vi "svx_Orbit SC Menu.vi"(6 "Run Mode?":bool, 7 "State":T2={"X Scale"={"Name"="Horizontal", "FString"="%#.2g", "Major Color"=16777238, "Minor Color"=16777216, "Scale Visible"=TRUE, " Label Visible"=TRUE, "Grid Style"=1}, "Y Scale"={"Name"="Vertical", "FString"="%#.2g", "Major Color"=16777238, "Minor Color"=16777216, "Scale Visible"=TRUE, " Label Visible"=TRUE, "Grid Style"=1}, "Plot"={"Point Style"=0, "Line Width"=0, "Line Style"=0, "Plot Color"=9727, "Point/fill"=0}, "Arrow/Crosshair Color"=9727, "Tacho Point Color"=16711680, "Container Bounds"={"Width"=563, "Height"=294}, "Axis Maximum"=10.0, "Probe Angles"={"Angle X"=0.0, "Angle Y"=1.5707963267948966}, "Background Color"=16777226, "Cursor"={"Cursor Point Style"=13, "Cursor Style"=4, "Cursor Line Width"=1, "Cursor Line Style"=0, "Cursor Color"=9727, "Cursor Name Visible"=TRUE, "Cursor Visible"=TRUE, "Cursor Position"={"X"=0.0, "Y"=0.0}, "Cursor Index"=0, "Cursor Lock"=FALSE}, "Elliptical Info"=[], "Legend Visible"=TRUE, "Scale Range Change"=refnum, "Strings[]"={"Custom pair name"=FALSE, "Row Strings []"=[], "Column Strings []"=[]}, "Index"=[{"pair index"=0, "order index"=0}], " Parents Tags"=[], "Children Tags"=[], "Open?"=[], "Label"="", "Legend Width"=120, "Pair Strings Changed?"=FALSE, "Size"=[], "Legend Background"=16777226, "Legend Font"=16777222, "Cursor Release"=refnum, "Autoscale"=TRUE, "Precession Direction"=[], "Item Width"=0, "User Pair Strings []"=[], "Users Order Strings []"=[], "Autoscale Once"=TRUE, "Property Write"=refnum} {"Index"."order index" min=0; "Index"."pair index" min=0; "Axis Maximum" min=0.0}, 10 "Refnum":refnum<vi>, 11 "MenuRef":refnum<k9>) -> ()   [LabVIEW 2017, in "SVX Orbit.xctl"]
uses:
  <vilib>/addons/_XControls/Orbit Plot/SVX Orbit.xctl
  <vilib>/addons/_XControls/Orbit Plot/subVIs/svx_Orbit Internal State.ctl
  <vilib>/addons/_XControls/Orbit Plot/subVIs/svx_Orbit Bounds.ctl
panel:
  in  "Run-time\nnew menu":T1(array[cluster])=[{"menu tag"="APP_SC_VISIBLE_ITEMS", "item names"="Plot Legend", "item tags"="USER_SC_SELECTOR", ""}, {"menu tag"="APP_SC_VISIBLE_ITEMS", "item names"="-", "item tags"="APP_SC_SEPERATOR_3", "USER_SC_SELECTOR"}, {"menu tag"="APP_SC_VISIBLE_ITEMS", "item names"="X Scale", "item tags"="USER_SC_X_SCALE", "APP_SC_SEPERATOR_3"}, {"menu tag"="APP_SC_VISIBLE_ITEMS", "item names"="Y Scale", "item tags"="USER_SC_Y_SCALE", "USER_SC_X_SCALE"}, {"menu tag"="APP_SC_VISIBLE_ITEMS", "item names"="-", "item tags"="APP_SC_SEPERATOR", "USER_SC_Y_SCALE"}, {"menu tag"="APP_SC_VISIBLE_ITEMS", "item names"="Cursor", "item tags"="USER_SC_CURSOR", "APP_SC_SEPERATOR"}, {"menu tag"="APP_SC_VISIBLE_ITEMS", "item names"="Cursor Info", "item tags"="USER_SC_CURSORINFO", "USER_SC_CURSOR"}, {"menu tag"="APP_SC_VISIBLE_ITEMS", "item names"="Lock Cursor Info Position", "item tags"="USER_SC_LOCK", "USER_SC_CURSORINFO"}, {"menu tag"="", "item names"="Autoscale", "item tags"="USER_SC_AUTOSCALE", ""}]
  in  "Edit-time\nnew menu":T1(array[cluster])=[{"menu tag"="USER_SC_VISIBLE_ITEMS", "item names"="Label", "item tags"="USER_SC_LABEL", ""}, {"menu tag"="USER_SC_VISIBLE_ITEMS", "item names"="Caption", "item tags"="USER_SC_CAPTION", "USER_SC_LABEL"}, {"menu tag"="USER_SC_VISIBLE_ITEMS", "item names"="-", "item tags"="APP_SC_SEPERATOR", "USER_SC_CAPTION"}, {"menu tag"="USER_SC_VISIBLE_ITEMS", "item names"="Plot Legend", "item tags"="USER_SC_SELECTOR", "APP_SC_SEPERATOR"}, {"menu tag"="USER_SC_VISIBLE_ITEMS", "item names"="-", "item tags"="APP_SC_SEPERATOR_3", "USER_SC_SELECTOR"}, {"menu tag"="USER_SC_VISIBLE_ITEMS", "item names"="X Scale", "item tags"="USER_SC_X_SCALE", "APP_SC_SEPERATOR_3"}, {"menu tag"="USER_SC_VISIBLE_ITEMS", "item names"="Y Scale", "item tags"="USER_SC_Y_SCALE", "USER_SC_X_SCALE"}, {"menu tag"="USER_SC_VISIBLE_ITEMS", "item names"="-", "item tags"="APP_SC_SEPERATOR_4", "USER_SC_Y_SCALE"}, {"menu tag"="USER_SC_VISIBLE_ITEMS", "item names"="Cursor", "item tags"="USER_SC_CURSOR", "APP_SC_SEPERATOR_4"}, {"menu tag"="USER_SC_VISIBLE_ITEMS", "item names"="Cursor Info", "item tags"="USER_SC_CURSORINFO", "USER_SC_CURSOR"}, {"menu tag"="USER_SC_VISIBLE_ITEMS", "item names"="Lock Cursor Info Position", "item tags"="USER_SC_LOCK", "USER_SC_CURSORINFO"}, {"menu tag"="", "item names"="Autoscale", "item tags"="USER_SC_AUTOSCALE", ""}, {"menu tag"="", "item names"="-", "item tags"="APP_SC_SEPERATOR_2", "USER_SC_AUTOSCALE"}, {"menu tag"="", "item names"="Properties", "item tags"="USER_SC_PROPERTIES", "APP_SC_SEPARATOR_2"}]
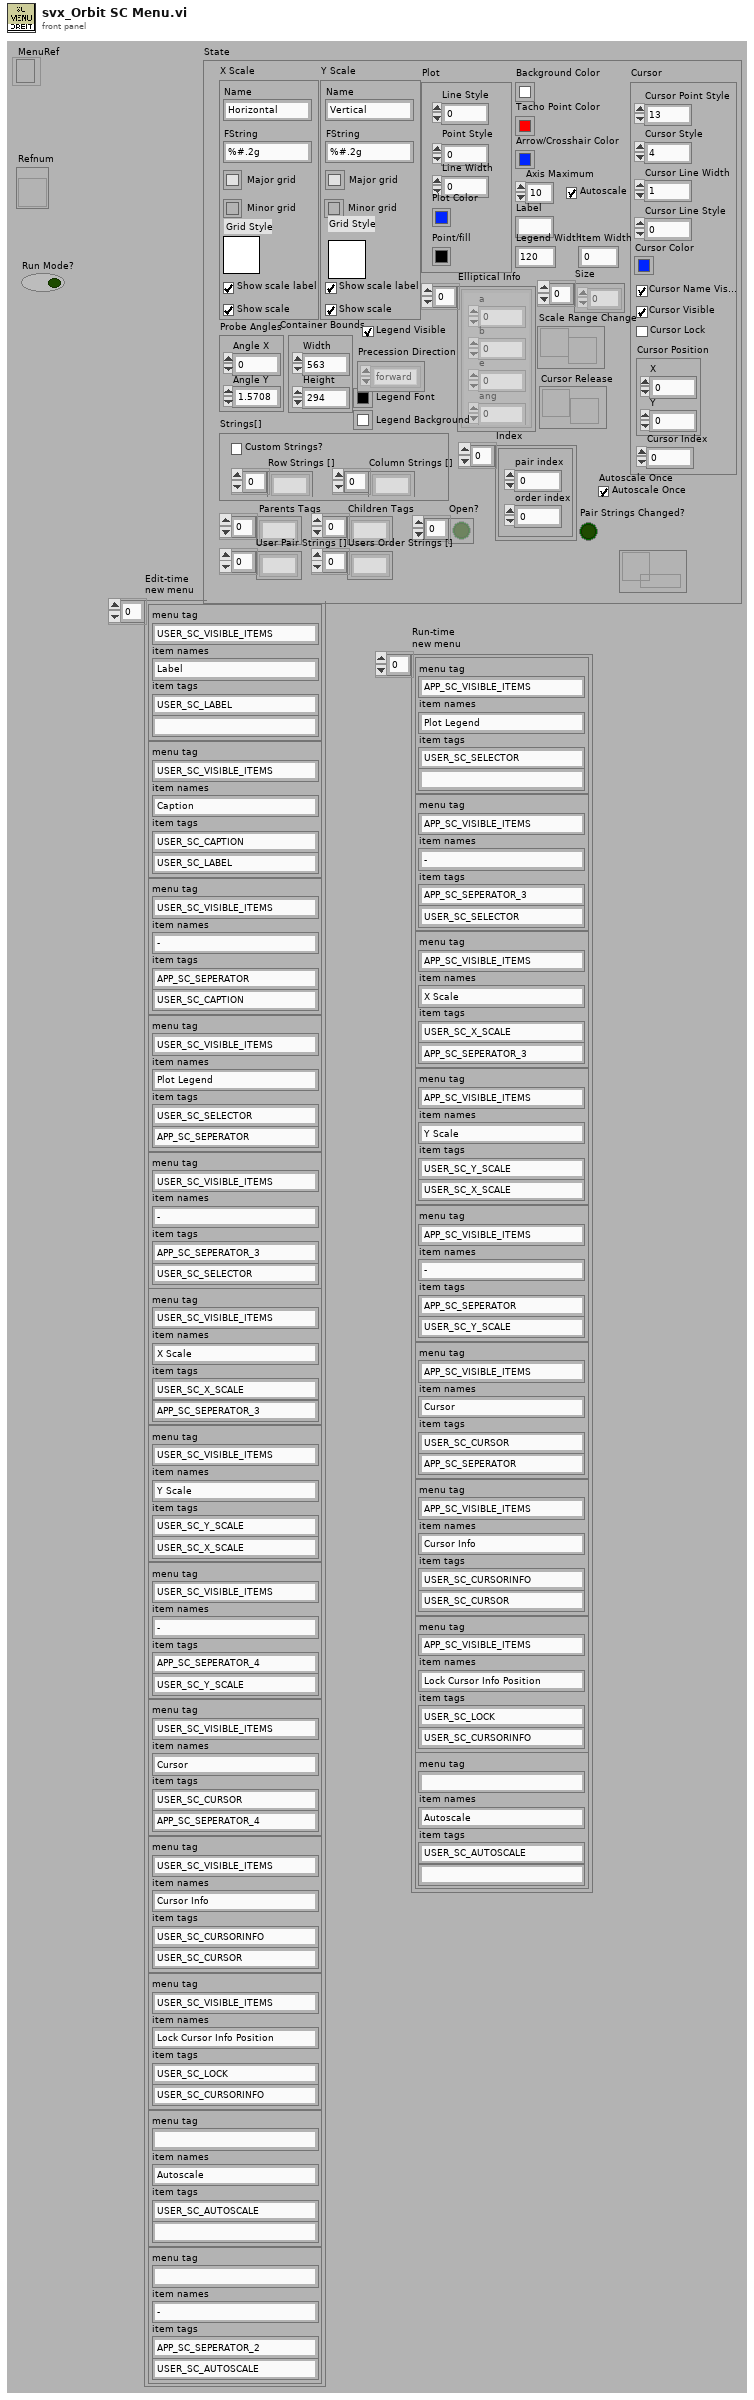
[diagram p1: front panel]
types:
  T1 = cluster{"menu tag":string, "item names":string, "item tags":string, string}[]
  T2 = typedef "SVX Orbit.xctl/svx_Orbit Internal State.ctl" = cluster{"X Scale":cluster{"Name":string, "FString":string, "Major Color":u32, "Minor Color":u32, "Scale Visible":bool, " Label Visible":bool, "Grid Style":u16}, "Y Scale":cluster{"Name":string, "FString":string, "Major Color":u32, "Minor Color":u32, "Scale Visible":bool, " Label Visible":bool, "Grid Style":u16}, "Plot":cluster{"Point Style":u8, "Line Width":u8, "Line Style":u8, "Plot Color":u32, "Point/fill":u32}, "Arrow/Crosshair Color":u32, "Tacho Point Color":u32, "Container Bounds":T3, "Axis Maximum":dbl, "Probe Angles":cluster{"Angle X":dbl, "Angle Y":dbl}, "Background Color":u32, "Cursor":cluster{"Cursor Point Style":u8, "Cursor Style":u8, "Cursor Line Width":u8, "Cursor Line Style":u8, "Cursor Color":u32, "Cursor Name Visible":bool, "Cursor Visible":bool, "Cursor Position":cluster{"X":dbl, "Y":dbl}, "Cursor Index":i32, "Cursor Lock":bool}, "Elliptical Info":cluster{"a":dbl, "b":dbl, "e":dbl, "ang":dbl}[], "Legend Visible":bool, "Scale Range Change":refnum<user-event>, "Strings[]":cluster{"Custom pair name":bool, "Row Strings []":string[], "Column Strings []":string[]}, "Index":cluster{"pair index":i32, "order index":i32}[], " Parents Tags":string[], "Children Tags":string[], "Open?":bool[], "Label":string, "Legend Width":u32, "Pair Strings Changed?":bool, "Size":i32[], "Legend Background":u32, "Legend Font":u32, "Cursor Release":refnum<user-event>, "Autoscale":bool, "Precession Direction":enum16{"forward", "backward"}[], "Item Width":u32, "User Pair Strings []":string[], "Users Order Strings []":string[], "Autoscale Once":bool, "Property Write":refnum<queue>}
  T3 = typedef "SVX Orbit.xctl/svx_Orbit Bounds.ctl" = cluster{"Width":u32, "Height":u32}
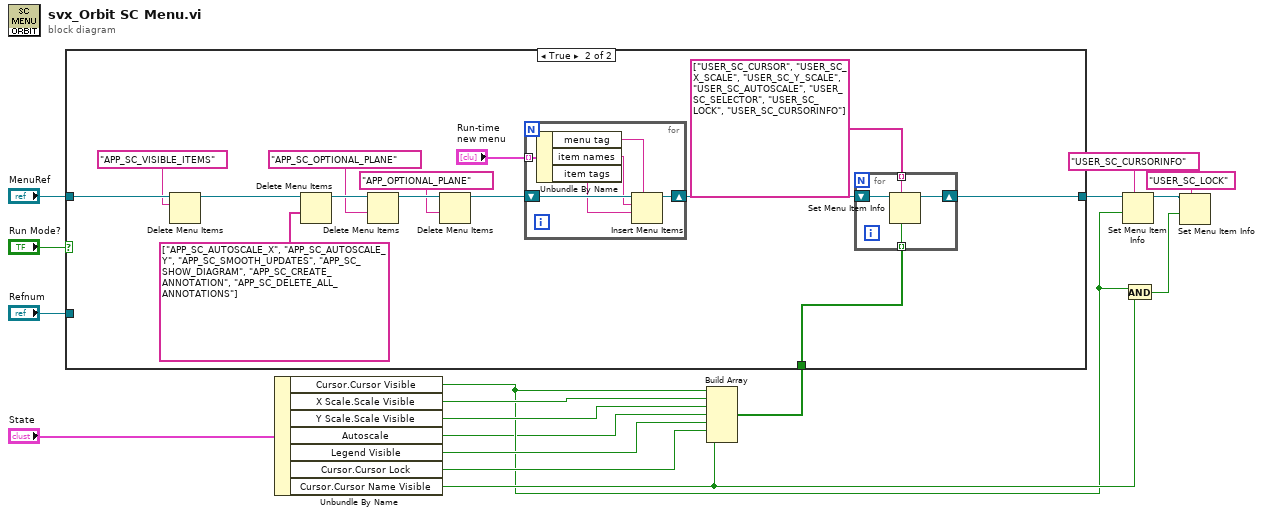
[diagram p0: block diagram]
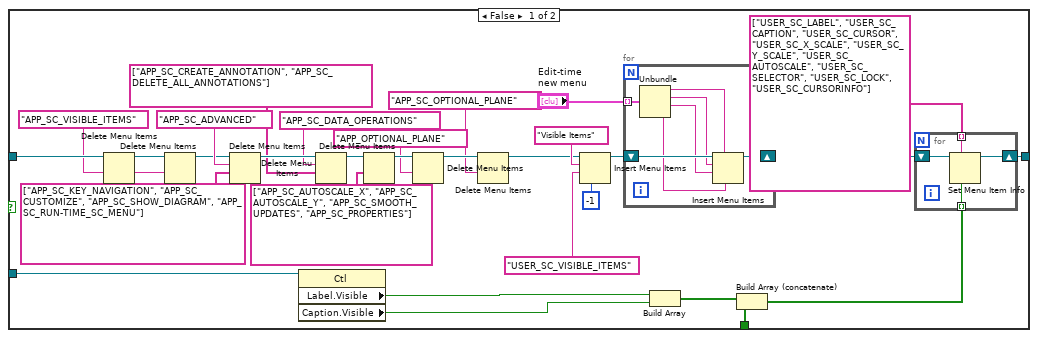
[diagram p2: hidden frame]
diagram:
  n1 = Unbundle By Name("State") -> ("Cursor.Cursor Visible"=w2:bool, "X Scale.Scale Visible"=w13:bool, "Y Scale.Scale Visible"=w12:bool, "Autoscale"=w1:bool, "Legend Visible"=w10:bool, "Cursor.Cursor Lock"=w9:bool, "Cursor.Cursor Name Visible"=w3:bool)
  n2 = Build Array(w2, w13, w12, w1, w10, w9, w3) -> (w11:bool[])
  n3 = case shown="True" "Run Mode?" {
    tunnel: "MenuRef" -> [w42 w72]
    tunnel: "Refnum" -> [w32 _]
    tunnel: w11 -> [w28 w65]
    tunnel: [w22 w64] -> w4
    frame False {
      w39 = "APP_SC_VISIBLE_ITEMS" ("menu tag")
      n4 = Delete Menu Items(7:w39, 9:w42) -> (3:w41:refnum<k9>)  [unwired: 2 in, 1 out]
      n5 = Delete Menu Items(7:w39, 9:w41) -> (3:w40:refnum<k9>)  [unwired: 2 in, 1 out]
      n6 = Delete Menu Items(7:string[] ["APP_SC_KEY_NAVIGATION", "APP_SC_CUSTOMIZE", "APP_SC_SHOW_DIAGRAM", "APP_SC_RUN-TIME_SC_MENU"], 8:"APP_SC_ADVANCED" ("menu tag"), 9:w40) -> (3:w26:refnum<k9>)  [unwired: 1 in, 1 out]
      n7 = property class="Ctl"(reference=w32) -> ("Label.Visible"=w31:bool, "Caption.Visible"=w30:bool)  [unwired: 1 in, 2 out]
      n8 = Delete Menu Items(7:string[] ["APP_SC_CREATE_ANNOTATION", "APP_SC_DELETE_ALL_ANNOTATIONS"], 8:"APP_SC_DATA_OPERATIONS" ("menu tag"), 9:w26) -> (3:w24:refnum<k9>)  [unwired: 1 in, 1 out]
      n9 = Delete Menu Items(7:string[] ["APP_SC_AUTOSCALE_X", "APP_SC_AUTOSCALE_Y", "APP_SC_SMOOTH_UPDATES", "APP_SC_PROPERTIES"], 9:w24) -> (3:w44:refnum<k9>)  [unwired: 2 in, 1 out]
      n10 = Delete Menu Items(7:"APP_OPTIONAL_PLANE" ("menu tag"), 9:w44) -> (3:w20:refnum<k9>)  [unwired: 2 in, 1 out]
      n11 = Delete Menu Items(7:"APP_SC_OPTIONAL_PLANE" ("menu tag"), 9:w20) -> (3:w19:refnum<k9>)  [unwired: 2 in, 1 out]
      n12 = Insert Menu Items(4:-1, 7:"USER_SC_VISIBLE_ITEMS", 8:"Visible Items" ("item names"), 9:w19) -> (3:w35:refnum<k9>)  [unwired: 2 in, 2 out]
      n13 = for {
        shift-right: [w57] -> w34
        shift-left: w35 -> [w58]
        tunnel: "Edit-time\nnew menu" -> [w56] mode=indexing
        n14 = Unbundle(w56) -> ("menu tag"=w55:string, "item names"=w54:string, "item tags"=w53:string, w52:string)
        n15 = Insert Menu Items(4:w52, 5:w55, 7:w53, 8:w54, 9:w58) -> (3:w57:refnum<k9>)  [unwired: 1 in, 2 out]
      }
      n16 = Build Array(w31, w30) -> (w29:bool[])
      n17 = Build Array (concatenate)(w29, w28) -> (w27:bool[])
      n18 = for {
        shift-right: [w50] -> w22
        shift-left: w34 -> [w51]
        tunnel: string[] ["USER_SC_LABEL", "USER_SC_CAPTION", "USER_SC_CURSOR", "USER_SC_X_SCALE", "USER_SC_Y_SCALE", "USER_SC_AUTOSCALE", "USER_SC_SELECTOR", "USER_SC_LOCK", "USER_SC_CURSORINFO"] ("item tags") -> [w49] mode=indexing
        tunnel: w27 -> [w48] mode=indexing
        n19 = Set Menu Item Info(6:w48, 7:w49, 11:w51) -> (3:w50:refnum<k9>)  [unwired: 4 in, 1 out]
      }
    }
    frame True {
      n20 = Delete Menu Items(8:"APP_SC_VISIBLE_ITEMS" ("menu tag"), 9:w72) -> (3:w71:refnum<k9>)  [unwired: 2 in, 1 out]
      n21 = Delete Menu Items(7:string[] ["APP_SC_AUTOSCALE_X", "APP_SC_AUTOSCALE_Y", "APP_SC_SMOOTH_UPDATES", "APP_SC_SHOW_DIAGRAM", "APP_SC_CREATE_ANNOTATION", "APP_SC_DELETE_ALL_ANNOTATIONS"], 9:w71) -> (3:w63:refnum<k9>)  [unwired: 2 in, 1 out]
      n22 = Delete Menu Items(7:"APP_SC_OPTIONAL_PLANE" ("menu tag"), 9:w63) -> (3:w61:refnum<k9>)  [unwired: 2 in, 1 out]
      n23 = Delete Menu Items(7:"APP_OPTIONAL_PLANE" ("menu tag"), 9:w61) -> (3:w60:refnum<k9>)  [unwired: 2 in, 1 out]
      n24 = for {
        tunnel: "Run-time\nnew menu" -> [w81] mode=indexing
        shift-right: [w77] -> w66
        shift-left: w60 -> [w82]
        n25 = Unbundle By Name(w81) -> ("menu tag"=w80:string, "item names"=w79:string, "item tags"=w78:string)
        n26 = Insert Menu Items(5:w80, 7:w78, 8:w79, 9:w82) -> (3:w77:refnum<k9>)  [unwired: 2 in, 2 out]
      }
      n27 = for {
        shift-right: [w75] -> w64
        shift-left: w66 -> [w76]
        tunnel: string[] ["USER_SC_CURSOR", "USER_SC_X_SCALE", "USER_SC_Y_SCALE", "USER_SC_AUTOSCALE", "USER_SC_SELECTOR", "USER_SC_LOCK", "USER_SC_CURSORINFO"] ("item tags") -> [w74] mode=indexing
        tunnel: w65 -> [w73] mode=indexing
        n28 = Set Menu Item Info(6:w73, 7:w74, 11:w76) -> (3:w75:refnum<k9>)  [unwired: 4 in, 1 out]
      }
    }
  }
  n29 = Set Menu Item Info(7:"USER_SC_CURSORINFO" ("String"), 9:w2, 11:w4) -> (3:w8:refnum<k9>)  [unwired: 4 in, 1 out]
  n30 = And(x=w2, y=w3) -> (x .and. y?=w5:bool)
  n31 = Set Menu Item Info(7:"USER_SC_LOCK" ("String"), 9:w5, 11:w8) -> ()  [unwired: 4 in, 2 out]
